vi "CommandPickup.vi"(9 "Gripper Value R":dbl, 10 "Gripper Value L":dbl, 11 "Elevator Value":dbl) -> (3 "appended array":cluster{"States":T1, "Numeric":dbl}[](array[cluster]))   [LabVIEW 2017]
uses:
  Typedef/TeirNumber.ctl
  Elevator/Private/Typedef/Sequencer States.ctl
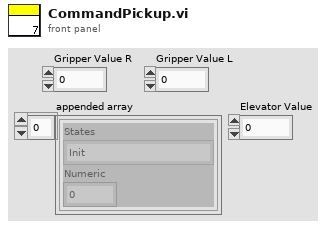
[diagram p1: front panel]
types:
  T1 = typedef "Sequencer States.ctl" = enum16{"Init", "Set Elevator SP", "Set Gripper SP", "Wait For Elevator", "Wait For Gripper", ""}
  T2 = typedef "TeirNumber.ctl" = enum16{"T1", "T2", "T3", "T4", "T5", "T6"}
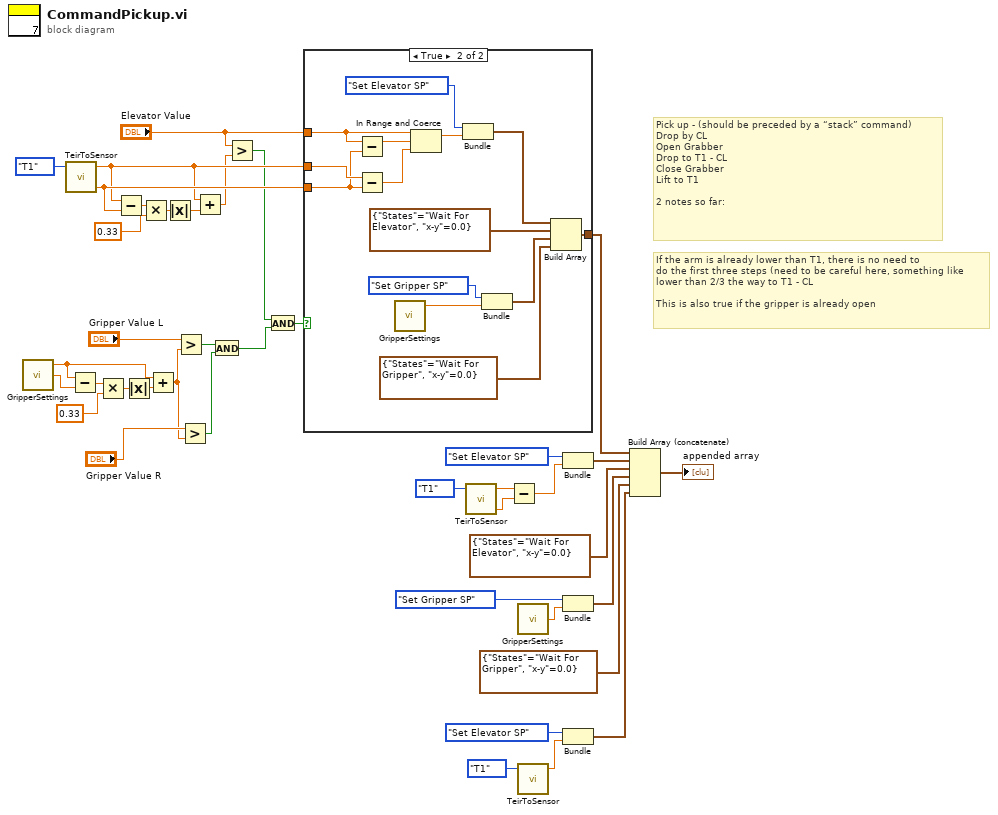
[diagram p0: block diagram]
diagram:
  # "If the arm is already lower than T1, there is no need to \ndo the first three steps (need to be careful here, something like \nlower than 2/3 the way to T1 - CL \n\nThis is also true if the gripper is already open"
  # "Pick up - (should be preceded by a “stack” command)\nDrop by CL\nOpen Grabber\nDrop to T1 - CL\nClose Grabber\nLift to T1\n\n2 notes so far:"
  n1 = call "GripperSettings.vi"() -> ("Open"=w12:dbl, "Close"=w7:dbl)  [unwired: 2 in, 1 out]
  n2 = call "TeirToSensor.vi"("Teir"=TeirNumber."T1" ("Enum")) -> ("CL"=w21:dbl, "Teir Height"=w17:dbl)  [unwired: 2 in, 1 out]
  n3 = Subtract(x=w12, y=w7) -> (x-y=w8:dbl)
  n4 = Multiply(x=w8, y=0.33) -> (x*y=w10:dbl)
  n5 = Subtract(x=w17, y=w21) -> (x-y=w20:dbl)
  n6 = Absolute Value(x=w10) -> (abs(x)=w11:dbl)
  n7 = Multiply(x=w20, y=0.33) -> (x*y=w18:dbl)
  n8 = Add(x=w12, y=w11) -> (x+y=w3:dbl)
  n9 = Absolute Value(x=w18) -> (abs(x)=w15:dbl)
  n10 = Greater?(x="Gripper Value L", y=w3) -> (0:w5:bool)
  n11 = Greater?(x="Gripper Value R", y=w3) -> (0:w2:bool)
  n12 = Add(x=w17, y=w15) -> (x+y=w16:dbl)
  n13 = And(x=w5, y=w2) -> (x .and. y?=w1:bool)
  n14 = Greater?(x="Elevator Value", y=w16) -> (0:w13:bool)
  n15 = And(x=w13, y=w1) -> (x .and. y?=w14:bool)
  n16 = case shown="True" w14 {
    tunnel: w17 -> [_ w52]
    tunnel: w21 -> [_ w51]
    tunnel: "Elevator Value" -> [_ w49]
    tunnel: [_ w43] -> w22
    frame False {
    }
    frame True {
      n17 = Subtract(x=w49, y=w51) -> (x-y=w53:dbl)
      n18 = Subtract(x=w52, y=w51) -> (x-y=w50:dbl)
      n19 = call "GripperSettings.vi"() -> ("Open"=w41:dbl)  [unwired: 2 in, 2 out]
      n20 = In Range and Coerce(upper limit=w49, x=w53, lower limit=w50) -> (coerced(x)=w48:dbl)  [unwired: 1 out]
      n21 = Bundle("States"=Sequencer_States."Set Elevator SP", "Elevator Value"=w48) -> (w47:cluster{"States":T1, "Elevator Value":dbl})  [unwired: 1 in]
      n22 = Bundle("States"=Sequencer_States."Set Gripper SP", "Open"=w41) -> (w45:cluster{"States":T1, "Open":dbl})  [unwired: 1 in]
      n23 = Build Array(w47, cluster{"States":T1, "x-y":dbl} {"States"=enum."Wait For Elevator", "x-y"=0.0}, w45, cluster{"States":T1, "x-y":dbl} {"States"=enum."Wait For Gripper", "x-y"=0.0}) -> (w43:cluster{"States":T1, "x-y":dbl}[])
    }
  }
  n24 = call "TeirToSensor.vi"("Teir"=TeirNumber."T1" ("Enum")) -> ("CL"=w35:dbl, "Teir Height"=w34:dbl)  [unwired: 2 in, 1 out]
  n25 = Subtract(x=w34, y=w35) -> (x-y=w32:dbl)
  n26 = call "GripperSettings.vi"() -> ("Close"=w27:dbl)  [unwired: 2 in, 2 out]
  n27 = call "TeirToSensor.vi"("Teir"=TeirNumber."T1" ("Enum")) -> ("Teir Height"=w37:dbl)  [unwired: 2 in, 2 out]
  n28 = Bundle("States"=Sequencer_States."Set Elevator SP", w32) -> (w30:cluster{"States":T1, dbl})  [unwired: 1 in]
  n29 = Bundle("States"=Sequencer_States."Set Gripper SP", "Close"=w27) -> (w28:cluster{"States":T1, "Close":dbl})  [unwired: 1 in]
  n30 = Bundle("States"=Sequencer_States."Set Elevator SP", "Teir Height"=w37) -> (w39:cluster{"States":T1, "Teir Height":dbl})  [unwired: 1 in]
  n31 = Build Array (concatenate)(w22, w30, cluster{"States":T1, "x-y":dbl} {"States"=enum."Wait For Elevator", "x-y"=0.0}, w28, cluster{"States":T1, "x-y":dbl} {"States"=enum."Wait For Gripper", "x-y"=0.0}, w39) -> (→"appended array":cluster{"States":T1, "Teir Height":dbl}[])
